vi "Advance past Number.vi"(7 "JSON":string, 9 "Offset (0)":i32, 11 "Parser State in":T2=enum."Number/Other") -> (1 "Offset past match":i32, 3 "Parser State":T2, 4 "JSON Value Type":T1, 6 "Value start out":i32)   [LabVIEW 2017, in "JSONtext.lvlib"]
uses:
  JSONtext.lvlib
  Parsing State.ctl
  JSON Value Type.ctl
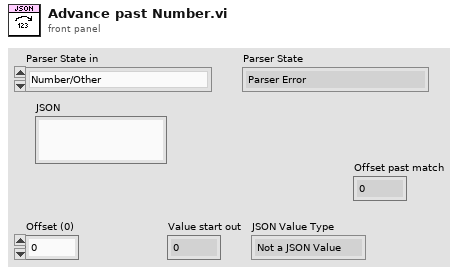
[diagram p1: front panel]
types:
  T1 = typedef "JSONtext.lvlib/JSON Value Type.ctl" = enum16{"Not a JSON Value", "JSON Object", "JSON Array", "String", "Number", "true", "false", "null"}
  T2 = typedef "JSONtext.lvlib/Parsing State.ctl" = enum16{"Parser Error", "Object", "Array", "String", "Number/Other", "Leading Whitespace", "Object end", "Array end", "Value end"}
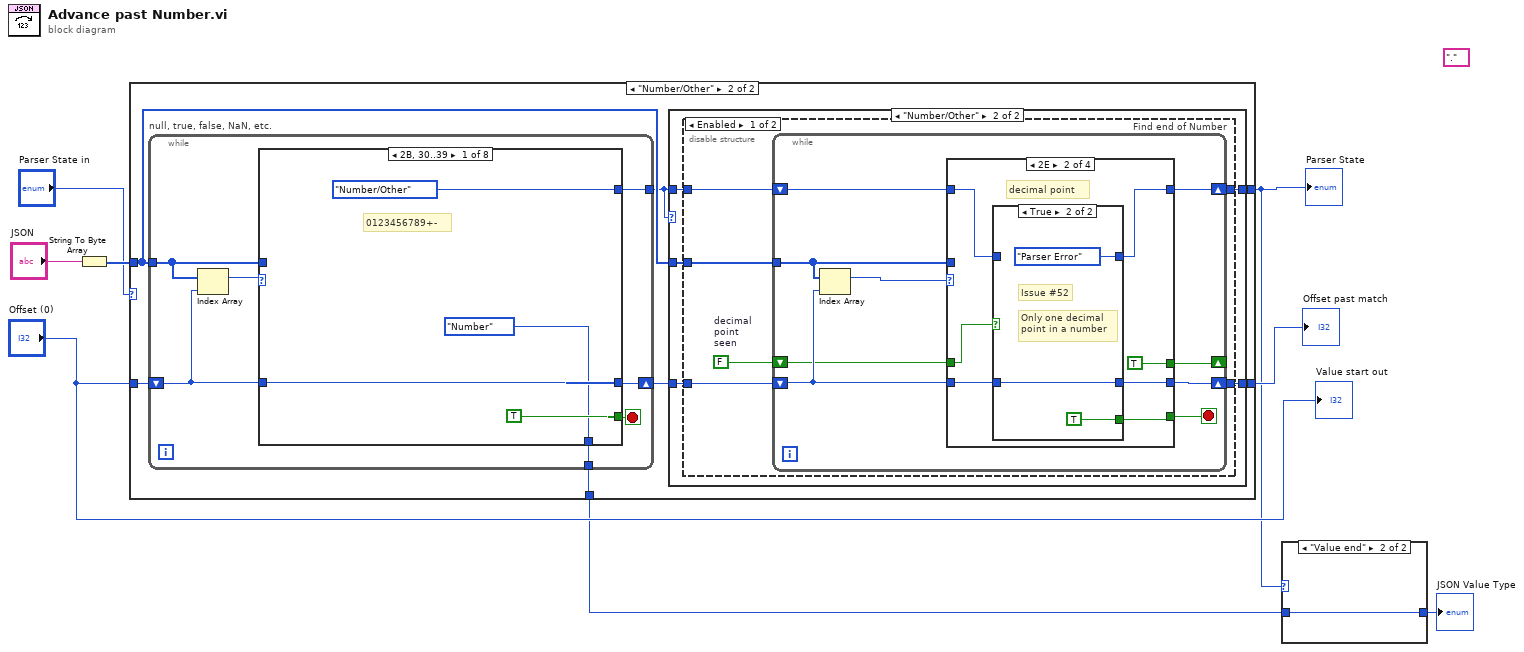
[diagram p0: block diagram]
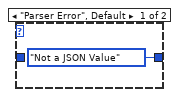
[diagram p2: hidden frame]
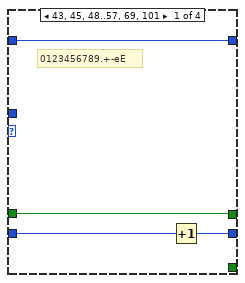
[diagram p5: hidden frame]
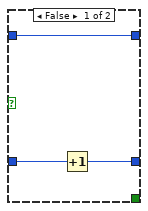
[diagram p6: hidden frame]
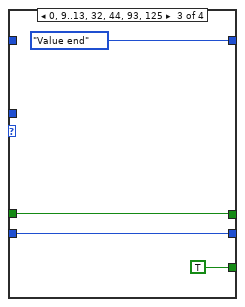
[diagram p7: hidden frame]
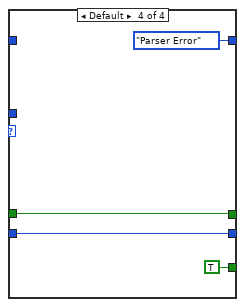
[diagram p8: hidden frame]
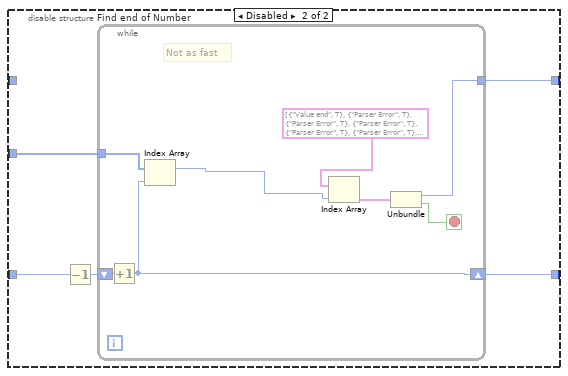
[diagram p9: hidden frame]
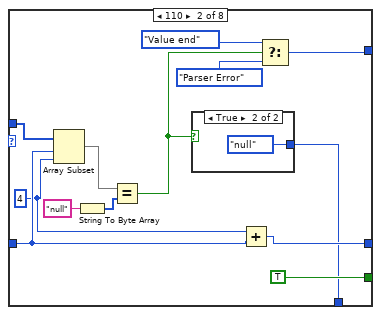
[diagram p10: hidden frame]
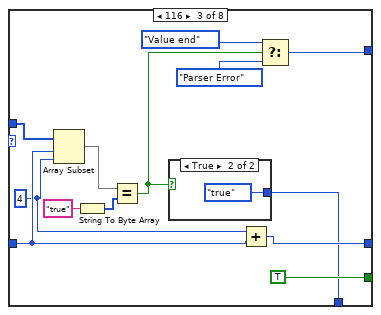
[diagram p12: hidden frame]
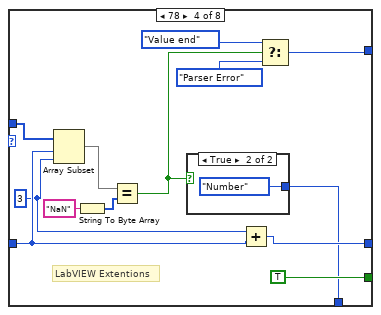
[diagram p14: hidden frame]
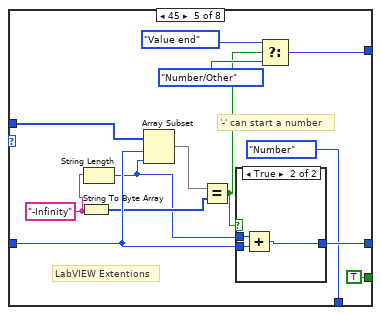
[diagram p16: hidden frame]
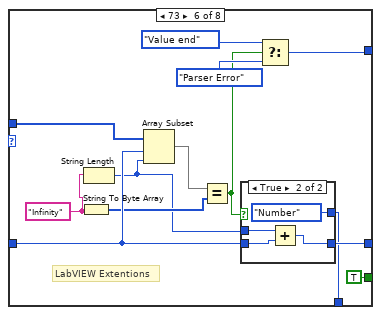
[diagram p18: hidden frame]
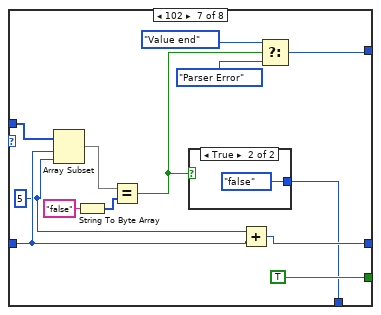
[diagram p20: hidden frame]
diagram:
  (unwired) "."
  n1 = String To Byte Array(string="JSON") -> (unsigned byte array=w5:u8[])
  n2 = case shown="\"Number/Other\"" "Parser State in" {
    tunnel: [_ w16] -> w3
    tunnel: [w9 w15] -> w8
    tunnel: w5 -> [_ w13]
    tunnel: "Offset (0)" -> [w9 w11]
    tunnel: [_ w10] -> w2
    frame "Parser Error", Default {
    }
    frame "Number/Other" {
      n3 = while "null, true, false, NaN, etc." {
        tunnel: w13 -> [w82]
        shift-right: [w78] -> w14
        shift-left: w11 -> [w79]
        tunnel: [w81] -> w12
        tunnel: [w77] -> w10
        stop <- w80 stop-if-true
        n4 = Index Array(array=w82, index=w79) -> (element=w83:u8)
        n5 = case shown="2B, 30..39" w83 {
          tunnel: w82 -> [_ w99 w113 w127 w142 w159 w176 _]
          tunnel: [Parsing_State."Number/Other" w96 w110 w124 w140 w157 w173 Parsing_State."Parser Error"] -> w81
          tunnel: [TRUE TRUE TRUE TRUE TRUE TRUE TRUE TRUE] -> w80
          tunnel: w79 -> [w85 w92 w106 w120 w136 w153 w169 w182]
          tunnel: [w85 w90 w104 w118 w135 w152 w167 w182] -> w78
          tunnel: [JSON_Value_Type."Number" w88 w102 w116 JSON_Value_Type."Number" w147 w165 JSON_Value_Type."Not a JSON Value"] -> w77
          frame 43, 48..57 {
            # "0123456789+-"
          }
          frame 110 {
            w91 = 4 ("length")
            n6 = Array Subset(array=w99, index=w92, length=w91) -> (w97:u8[])
            n7 = String To Byte Array(string="null") -> (unsigned byte array=w98:u8[])
            n8 = Equal?(x=w97, y=w98) -> (x = y?=w89:bool)
            n9 = case shown="True" w89 {
              tunnel: [_ JSON_Value_Type."null"] -> w88
              frame False {
              }
              frame True {
              }
            }
            n10 = Add(x=w91, y=w92) -> (x+y=w90:i32)
            n11 = Select(t=Parsing_State."Value end", s=w89, f=Parsing_State."Parser Error") -> (s? t:f=w96:T2)
          }
          frame 116 {
            w105 = 4 ("length")
            n12 = Array Subset(array=w113, index=w106, length=w105) -> (w111:u8[])
            n13 = String To Byte Array(string="true") -> (unsigned byte array=w112:u8[])
            n14 = Equal?(x=w111, y=w112) -> (x = y?=w103:bool)
            n15 = case shown="True" w103 {
              tunnel: [_ JSON_Value_Type."true"] -> w102
              frame False {
              }
              frame True {
              }
            }
            n16 = Add(x=w105, y=w106) -> (x+y=w104:i32)
            n17 = Select(t=Parsing_State."Value end", s=w103, f=Parsing_State."Parser Error") -> (s? t:f=w110:T2)
          }
          frame 78 {
            w119 = 3 ("length")
            # "LabVIEW Extentions"
            n18 = Array Subset(array=w127, index=w120, length=w119) -> (w125:u8[])
            n19 = String To Byte Array(string="NaN") -> (unsigned byte array=w126:u8[])
            n20 = Equal?(x=w125, y=w126) -> (x = y?=w117:bool)
            n21 = case shown="True" w117 {
              tunnel: [_ JSON_Value_Type."Number"] -> w116
              frame False {
              }
              frame True {
              }
            }
            n22 = Add(x=w119, y=w120) -> (x+y=w118:i32)
            n23 = Select(t=Parsing_State."Value end", s=w117, f=Parsing_State."Parser Error") -> (s? t:f=w124:T2)
          }
          frame 45 {
            w133 = "-Infinity"
            # "'-' can start a number"
            # "LabVIEW Extentions"
            n24 = String To Byte Array(string=w133) -> (unsigned byte array=w134:u8[])
            n25 = String Length(string=w133) -> (length=w132:i32)
            n26 = Array Subset(array=w142, index=w136, length=w132) -> (w141:u8[])
            n27 = Equal?(x=w141, y=w134) -> (x = y?=w131:bool)
            n28 = case shown="True" w131 {
              tunnel: w136 -> [w143 w146]
              tunnel: [w143 w145] -> w135
              tunnel: w132 -> [_ w144]
              frame False {
              }
              frame True {
                n29 = Add(x=w144, y=w146) -> (x+y=w145:i32)
              }
            }
            n30 = Select(t=Parsing_State."Value end", s=w131, f=Parsing_State."Number/Other") -> (s? t:f=w140:T2)
          }
          frame 73 {
            w150 = "Infinity"
            # "LabVIEW Extentions"
            n31 = String To Byte Array(string=w150) -> (unsigned byte array=w151:u8[])
            n32 = String Length(string=w150) -> (length=w149:i32)
            n33 = Array Subset(array=w159, index=w153, length=w149) -> (w158:u8[])
            n34 = Equal?(x=w158, y=w151) -> (x = y?=w148:bool)
            n35 = case shown="True" w148 {
              tunnel: w153 -> [w160 w164]
              tunnel: [w160 w163] -> w152
              tunnel: w149 -> [_ w162]
              tunnel: [_ JSON_Value_Type."Number"] -> w147
              frame False {
              }
              frame True {
                n36 = Add(x=w162, y=w164) -> (x+y=w163:i32)
              }
            }
            n37 = Select(t=Parsing_State."Value end", s=w148, f=Parsing_State."Parser Error") -> (s? t:f=w157:T2)
          }
          frame 102 {
            w168 = 5 ("length")
            n38 = Array Subset(array=w176, index=w169, length=w168) -> (w174:u8[])
            n39 = String To Byte Array(string="false") -> (unsigned byte array=w175:u8[])
            n40 = Equal?(x=w174, y=w175) -> (x = y?=w166:bool)
            n41 = case shown="True" w166 {
              tunnel: [_ JSON_Value_Type."false"] -> w165
              frame False {
              }
              frame True {
              }
            }
            n42 = Add(x=w168, y=w169) -> (x+y=w167:i32)
            n43 = Select(t=Parsing_State."Value end", s=w166, f=Parsing_State."Parser Error") -> (s? t:f=w173:T2)
          }
          frame Default {
          }
        }
      }
      n44 = case shown="\"Number/Other\"" w12 {
        tunnel: [w17 w23] -> w16
        tunnel: [w18 w22] -> w15
        tunnel: w14 -> [w18 w19]
        tunnel: w12 -> [w17 w21]
        tunnel: w13 -> [_ w20]
        frame "Parser Error", Default {
        }
        frame "Number/Other" {
          n45 = disable-structure shown="Enabled" {
            disable-tunnel: [w29 w68] -> w23
            disable-tunnel: [w28 w67] -> w22
            disable-tunnel: w21 -> [w27 _]
            disable-tunnel: w20 -> [w26 w66]
            disable-tunnel: w19 -> [w25 w65]
            frame Enabled {
              w24 = FALSE  # decimal point seen
              n46 = while "Find end of Number" {
                tunnel: w26 -> [w38]
                shift-right: [w34] -> w28
                shift-left: w25 -> [w32]
                shift-right: [w36] -> w29
                shift-left: w27 -> [w37]
                shift-right: [w31] -> _
                shift-left: w24 -> [w30]
                stop <- w35 stop-if-true
                n47 = Index Array(array=w38, index=w32) -> (element=w33:u8)
                n48 = case shown="2E" w33 {
                  tunnel: w38 -> [_ _ _ _]
                  tunnel: w37 -> [w42 w45 _ _]
                  tunnel: [w42 w44 Parsing_State."Value end" Parsing_State."Parser Error"] -> w36
                  tunnel: [_ w43 TRUE TRUE] -> w35
                  tunnel: w32 -> [w41 w49 w57 w63]
                  tunnel: [w40 w48 w57 w63] -> w34
                  tunnel: [w39 TRUE w56 w60] -> w31
                  tunnel: w30 -> [w39 w46 w56 w60]
                  frame 43, 45, 48..57, 69, 101 {
                    # "0123456789.+-eE"
                    n49 = Increment(x=w41) -> (x+1=w40:i32)
                  }
                  frame 46 {
                    # "decimal point"
                    n50 = case shown="True" w46 {
                      tunnel: w49 -> [w52 w54]
                      tunnel: [w51 w54] -> w48
                      tunnel: [w50 Parsing_State."Parser Error"] -> w44
                      tunnel: w45 -> [w50 _]
                      tunnel: [_ TRUE] -> w43
                      frame False {
                        n51 = Increment(x=w52) -> (x+1=w51:i32)
                      }
                      frame True {
                        # "Only one decimal\npoint in a number"
                        # "Issue #52"
                      }
                    }
                  }
                  frame 0, 9..13, 32, 44, 93, 125 {
                  }
                  frame Default {
                  }
                }
              }
            }
            frame Disabled {
              n52 = Decrement(x=w65) -> (x-1=w64:i32)
              n53 = while "Find end of Number" {
                tunnel: w66 -> [w76]
                shift-right: [w69] -> w67
                shift-left: w64 -> [w75]
                tunnel: [w70] -> w68
                stop <- w71 stop-if-true
                # "Not as fast"
                n54 = Increment(x=w75) -> (x+1=w69:i32)
                n55 = Index Array(array=w76, index=w69) -> (element=w72:u8)
                n56 = Index Array(array=cluster{T2, bool}[] [{enum."Value end", TRUE}, {enum."Parser Error", TRUE}, {enum."Parser Error", TRUE}, {enum."Parser Error", TRUE}, {enum."Parser Error", TRUE}, {enum."Parser Error", TRUE}, {enum."Parser Error", TRUE}, {enum."Parser Error", TRUE}, {enum."Parser Error", TRUE}, {enum."Value end", TRUE}, {enum."Value end", TRUE}, {enum."Value end", TRUE}, {enum."Value end", TRUE}, {enum."Value end", TRUE}, {enum."Parser Error", TRUE}, {enum."Parser Error", TRUE}, {enum."Parser Error", TRUE}, {enum."Parser Error", TRUE}, {enum."Parser Error", TRUE}, {enum."Parser Error", TRUE}, {enum."Parser Error", TRUE}, {enum."Parser Error", TRUE}, {enum."Parser Error", TRUE}, {enum."Parser Error", TRUE}, {enum."Parser Error", TRUE}, {enum."Parser Error", TRUE}, {enum."Parser Error", TRUE}, {enum."Parser Error", TRUE}, {enum."Parser Error", TRUE}, {enum."Parser Error", TRUE}, {enum."Parser Error", TRUE}, {enum."Parser Error", TRUE}, {enum."Value end", TRUE}, {enum."Parser Error", TRUE}, {enum."Parser Error", TRUE}, {enum."Parser Error", TRUE}, {enum."Parser Error", TRUE}, {enum."Parser Error", TRUE}, {enum."Parser Error", TRUE}, {enum."Parser Error", TRUE}, {enum."Parser Error", TRUE}, {enum."Parser Error", TRUE}, {enum."Parser Error", TRUE}, {enum."Number/Other", FALSE}, {enum."Value end", TRUE}, {enum."Number/Other", FALSE}, {enum."Number/Other", FALSE}, {enum."Parser Error", TRUE}, {enum."Number/Other", FALSE}, {enum."Number/Other", FALSE}, {enum."Number/Other", FALSE}, {enum."Number/Other", FALSE}, {enum."Number/Other", FALSE}, {enum."Number/Other", FALSE}, {enum."Number/Other", FALSE}, {enum."Number/Other", FALSE}, {enum."Number/Other", FALSE}, {enum."Number/Other", FALSE}, {enum."Parser Error", TRUE}, {enum."Parser Error", TRUE}, {enum."Parser Error", TRUE}, {enum."Parser Error", TRUE}, {enum."Parser Error", TRUE}, {enum."Parser Error", TRUE}, {enum."Parser Error", TRUE}, {enum."Parser Error", TRUE}, {enum."Parser Error", TRUE}, {enum."Parser Error", TRUE}, {enum."Parser Error", TRUE}, {enum."Number/Other", FALSE}, {enum."Parser Error", TRUE}, {enum."Parser Error", TRUE}, {enum."Parser Error", TRUE}, {enum."Parser Error", TRUE}, {enum."Parser Error", TRUE}, {enum."Parser Error", TRUE}, {enum."Parser Error", TRUE}, {enum."Parser Error", TRUE}, {enum."Parser Error", TRUE}, {enum."Parser Error", TRUE}, {enum."Parser Error", TRUE}, {enum."Parser Error", TRUE}, {enum."Parser Error", TRUE}, {enum."Parser Error", TRUE}, {enum."Parser Error", TRUE}, {enum."Parser Error", TRUE}, {enum."Parser Error", TRUE}, {enum."Parser Error", TRUE}, {enum."Parser Error", TRUE}, {enum."Parser Error", TRUE}, {enum."Parser Error", TRUE}, {enum."Parser Error", TRUE}, {enum."Parser Error", TRUE}, {enum."Value end", TRUE}, {enum."Parser Error", TRUE}, {enum."Parser Error", TRUE}, {enum."Parser Error", TRUE}, {enum."Parser Error", TRUE}, {enum."Parser Error", TRUE}, {enum."Parser Error", TRUE}, {enum."Parser Error", TRUE}, {enum."Number/Other", FALSE}, {enum."Parser Error", TRUE}, {enum."Parser Error", TRUE}, {enum."Parser Error", TRUE}, {enum."Parser Error", TRUE}, {enum."Parser Error", TRUE}, {enum."Parser Error", TRUE}, {enum."Parser Error", TRUE}, {enum."Parser Error", TRUE}, {enum."Parser Error", TRUE}, {enum."Parser Error", TRUE}, {enum."Parser Error", TRUE}, {enum."Parser Error", TRUE}, {enum."Parser Error", TRUE}, {enum."Parser Error", TRUE}, {enum."Parser Error", TRUE}, {enum."Parser Error", TRUE}, {enum."Parser Error", TRUE}, {enum."Parser Error", TRUE}, {enum."Parser Error", TRUE}, {enum."Parser Error", TRUE}, {enum."Parser Error", TRUE}, {enum."Parser Error", TRUE}, {enum."Parser Error", TRUE}, {enum."Value end", TRUE}] ("Array"), index=w72) -> (element=w73:cluster{T2, bool})
                n57 = Unbundle(w73) -> (w70:T2, w71:bool)
              }
            }
          }
        }
      }
    }
  }
  "Parser State" <- w3
  "Offset past match" <- w8
  n58 = case shown="\"Value end\"" w3 {
    tunnel: w2 -> [_ w184]
    tunnel: [JSON_Value_Type."Not a JSON Value" w184] -> w1
    frame "Parser Error", Default {
    }
    frame "Value end" {
    }
  }
  "JSON Value Type" <- w1
  "Value start out" <- "Offset (0)"
